vi "DecodeVersionString.vi"(9 "VersionStr":string) -> (0 "build":i32, 1 "correction":i32, 2 "secondary":i32, 3 "Main":i32)   [LabVIEW 2015]
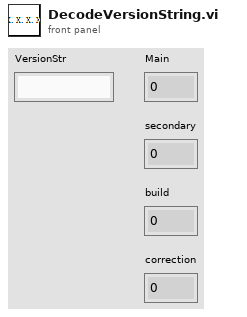
[diagram p1: front panel]
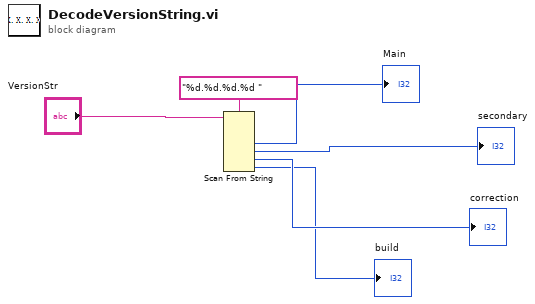
[diagram p0: block diagram]
diagram:
  n1 = Scan From String(format string="%d.%d.%d.%d " ("格式字符串"), input string="VersionStr") -> (output 1=→"Main":i32, output 2=→"secondary":i32, output 3=→"correction":i32, output 4=→"build":i32)  [unwired: 6 in, 3 out]
